vi "Bind Real.vi"(8 "error in (no error)":errorcluster, 10 "Real (DBL)":dbl, 11 "SQL Statement in":refnum<class "SQL Statement.lvclass">) -> (0 "error out":errorcluster, 3 "SQL Statement out":refnum<class "SQL Statement.lvclass">)   [LabVIEW 2023, in "SQLiteSupport.lvlib" / "SQL Statement.lvclass"]
doc: "Binds the next parameter as an SQLite3 REAL datatype (equivalent to a DBL)."
uses:
  SQL Statement.lvclass
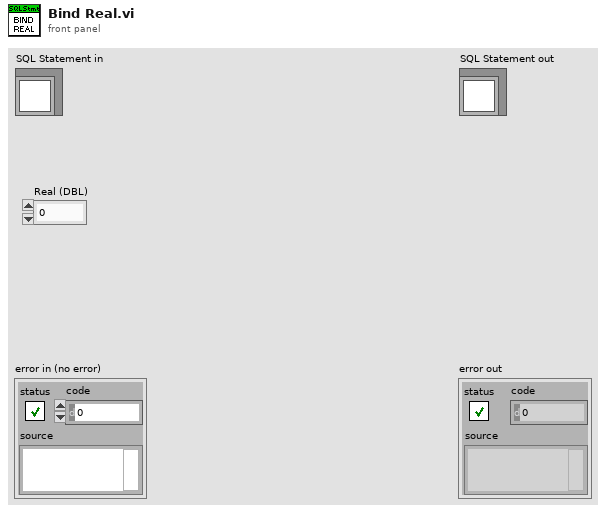
[diagram p1: front panel]
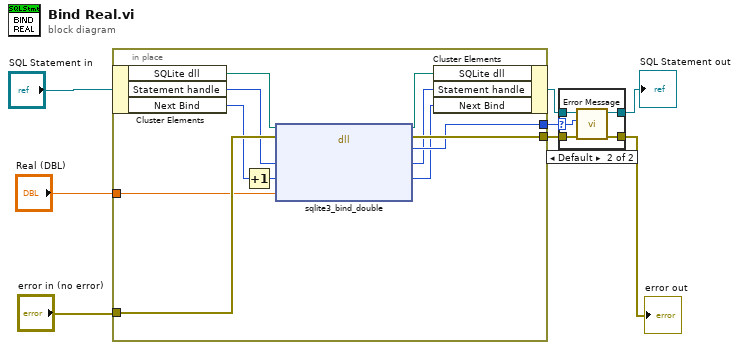
[diagram p0: block diagram]
diagram:
  n1 = in-place {
    in-place-border: "error in (no error)" -> [w19]
    in-place-border: "Real (DBL)" -> [w18]
    in-place-border: [w17] -> w6
    in-place-border: [w16] -> w5
    n2 = in-place-cluster #1("SQL Statement in") -> ("SQLite dll"=w14:path, "Statement handle"=w13:u64, "Next Bind"=w10:i32)
    n3 = Increment(x=w10) -> (x+1=w11:i32)
    n4 = dll-call lib="C:/LabVIEW_JDP/Support/SQLite/sqlite3.dll" fn="sqlite3_bind_double"(path in=w14, error in=w19, "Statement"=w13, "Parameter"=w11, "Real"=w18) -> (path out=w15:path, error out=w17:errorcluster, "Result Code"=w16:i32, "Statement"=w12:u64, "Parameter"=w9:i32)  [unwired: 2 in]
    n5 = in-place-cluster #1("SQLite dll"=w15, "Statement handle"=w12, "Next Bind"=w9) -> (w1:refnum<class "SQL Statement.lvclass">)
  }
  n6 = case shown="Default" w5 {
    selector: w5 -> [_ w23]
    tunnel: [w20 w26] -> w4
    tunnel: w6 -> [w21 w25]
    tunnel: [w21 w24] -> w3
    tunnel: w1 -> [w20 w22]
    frame 0 {
      # "No Error"
    }
    frame Default {
      n7 = call "Error Message.vi"("error in (no error)"=w25, "error code"=w23, "SQL Statement In"=w22) -> ("error out"=w24:errorcluster, "SQL Statement Out"=w26:refnum<class "SQL Statement.lvclass">)  [unwired: 7 in]
    }
  }
  "error out" <- w3
  "SQL Statement out" <- w4
